vi "Dynamic MFC Test.vi"() -> ()   [LabVIEW 2013]
doc: "This VI generates a square wave input and sends it to one of the MFCs for testing its dynamic response from zero."
uses:
  <vilib>/DAQmx/write.llb/DAQmx Write (Digital 1D Bool NChan 1Samp 1Line).vi
  <vilib>/DAQmx/write.llb/DAQmx Write (Analog 1D DBL NChan 1Samp).vi
  <vilib>/DAQmx/miscellaneous.llb/DAQmx Fill In Error Info.vi
  <vilib>/gmath/NI_Gmath.lvlib
panel:
  out "Input Signal":T1(graph)
  in  "Stop Button":bool
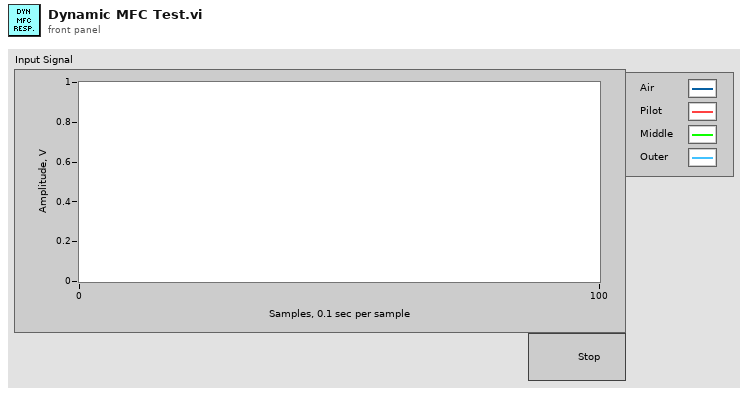
[diagram p1: front panel]
types:
  T1 = cluster{"[0]":dbl, "[1]":dbl, "[2]":dbl, "[3]":dbl, "[4]":dbl, "[5]":dbl, "[6]":dbl, "[7]":dbl, "[8]":dbl}
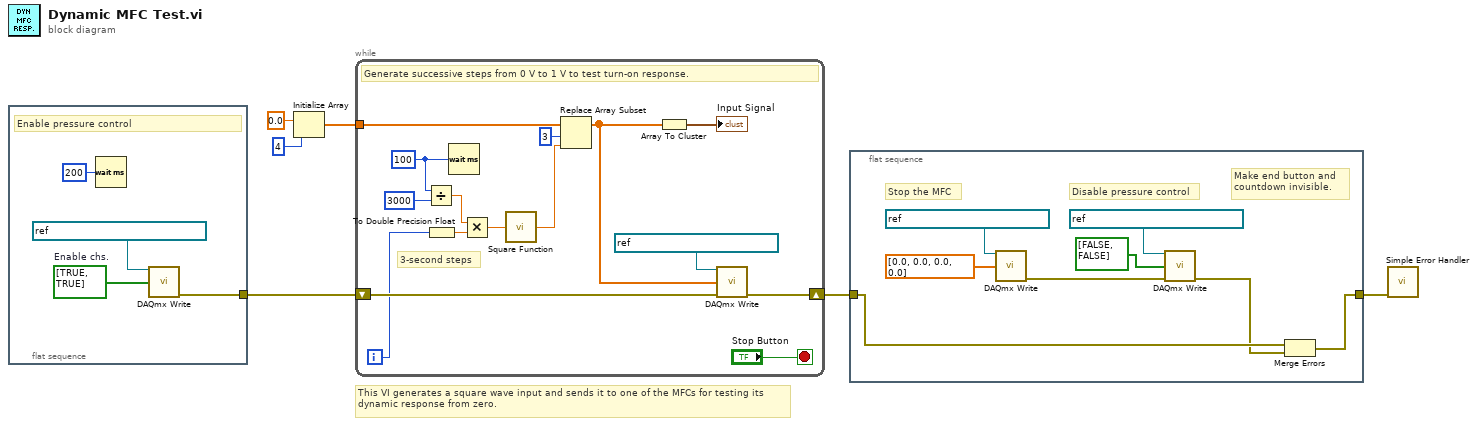
[diagram p0: block diagram]
diagram:
  # "This VI generates a square wave input and sends it to one of the MFCs for testing its dynamic response from zero."
  n1 = flat-sequence {
    tunnel: [w8] -> w6
    frame #0 {
      w7 = bool[] [TRUE, TRUE]  # Enable chs.
      # "Enable pressure control"
      n2 = Wait (ms)(milliseconds to wait=u32 200) -> ()  [unwired: 1 out]
      n3 = call-poly <vilib>:"DAQmx Write.vi"("task/channels in"=refnum<k21> "MFCOutputEnable_S2P0L67", "data"=w7) -> ("error out"=w8:errorcluster)  [unwired: 11 in, 2 out]
    }
  }
  n4 = Initialize Array(0.0 ("element"), 4 ("dimension size")) -> (w1:dbl[])
  n5 = while {
    shift-right: [w24] -> w5
    shift-left: w6 -> [w23]
    tunnel: w1 -> [w14]
    i -> [w21]
    stop <- "Stop Button" stop-if-true
    w20 = u32 100 ("milliseconds to wait")
    # "3-second steps"
    # "Generate successive steps from 0 V to 1 V to test turn-on response."
    n6 = Divide(x=w20, y=u32 3000) -> (x/y=w16:dbl)
    n7 = To Double Precision Float(number=w21) -> (double precision float=w18:dbl)
    n8 = Wait (ms)(milliseconds to wait=w20) -> ()  [unwired: 1 out]
    n9 = Multiply(x=w16, y=w18) -> (x*y=w15:dbl)
    n10 = call <vilib>:"Square Function.vi"("x"=w15) -> ("square(x)"=w13:dbl)
    n11 = Replace Array Subset(array=w14, new element=w13, index=3) -> (w11:dbl[])
    n12 = Array To Cluster(array=w11) -> (cluster=→"Input Signal":T1)
    n13 = call-poly <vilib>:"DAQmx Write.vi"("task/channels in"=refnum<k21> "MFCVoltageOut_S2AO0-3", "data"=w11, "error in"=w23) -> ("error out"=w24:errorcluster)  [unwired: 10 in, 2 out]
  }
  n14 = flat-sequence {
    tunnel: w5 -> [w29]
    tunnel: [w27] -> w4
    frame #0 {
      # "Make end button and\ncountdown invisible."
      # "Stop the MFC"
      # "Disable pressure control"
      n15 = call-poly <vilib>:"DAQmx Write.vi"("task/channels in"=refnum<k21> "MFCVoltageOut_S2AO0-3", "data"=dbl[] [0.0, 0.0, 0.0, 0.0]) -> ("error out"=w30:errorcluster)  [unwired: 11 in, 2 out]
      n16 = call-poly <vilib>:"DAQmx Write.vi"("task/channels in"=refnum<k21> "MFCOutputEnable_S2P0L67", "data"=bool[] [FALSE, FALSE], "error in"=w30) -> ("error out"=w28:errorcluster)  [unwired: 10 in, 2 out]
      n17 = Merge Errors(w29, w28) -> (w27:errorcluster)
    }
  }
  n18 = call <vilib>:"Simple Error Handler.vi"("error in (no error)"=w4) -> ()  [unwired: 4 in, 5 out]
